vi "Test TDMS.vi"() -> ()   [LabVIEW 2020]
uses:
  Models/Data Types/TDMS/TDMS.lvclass
  Models/Data Types/Abstrut Data/Abstruct Data Type.lvclass/Abstruct Data Type.ctl
  Models/Data Types/Abstrut Data/Accessors/Write File Path.vi
panel:
  in  "Horizontal Pointer Slide 3":cluster{"Numeric":dbl, "Numeric":dbl}(slide)={"Numeric"=0.0, "Numeric"=4.769230769230769} scale=0.0..10.0
  in  "Horizontal Pointer Slide 2":dbl(slide) scale=0.0..10.0
  in  "Horizontal Pointer Slide":cluster{"Numeric":dbl, "Numeric":dbl}(slide)={"Numeric"=0.0, "Numeric"=5.461538461538462} scale=0.0..10.0
  out "Waveform Chart":waveform(dbl)[](graph)
  out "error out":errorcluster
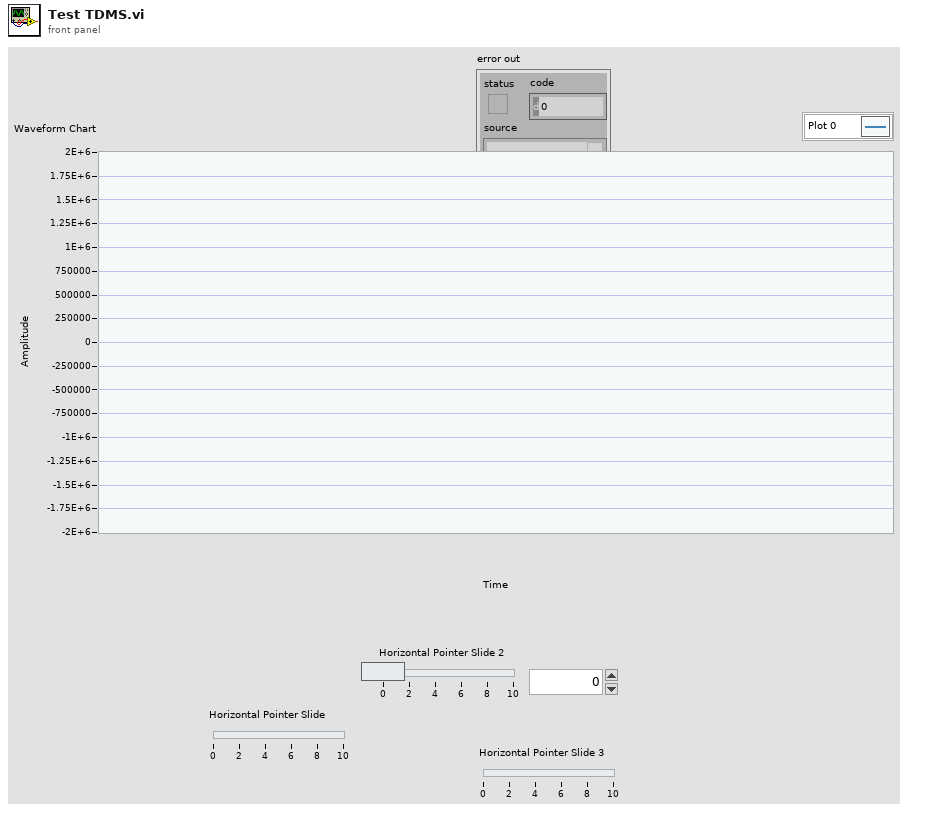
[diagram p1: front panel]
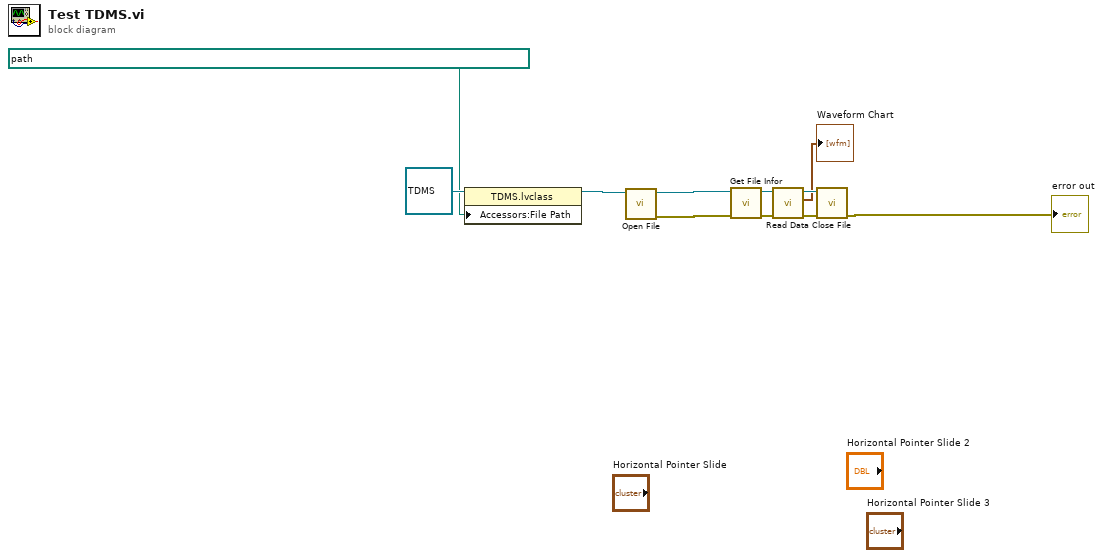
[diagram p0: block diagram]
diagram:
  n1 = property class="TDMS.lvclass"(reference=refnum<class "TDMS.lvclass"> refnum ("TDMS.lvclass"), "Accessors:File Path"=path "D:/13.软件工具/Data View/Source/Test Data/13 Calculate 2022-12-05 15-53-08.629.tdms" ("file path")) -> (reference out=w2:refnum<class "TDMS.lvclass">)  [unwired: 1 in, 1 out]
  n2 = call-dynamic "Open File.vi"("TDMS in"=w2) -> ("error out"=w10:errorcluster, "TDMS out"=w11:refnum<class "TDMS.lvclass">)  [unwired: 9 in]
  n3 = call-dynamic "Get File Infor.vi"("error in (no error)"=w10, "TDMS in"=w11) -> ("error out"=w8:errorcluster, "TDMS out"=w9:refnum<class "TDMS.lvclass">)  [unwired: 8 in]
  n4 = call-dynamic "Read Data.vi"("error in (no error)"=w8, "TDMS in"=w9) -> ("error out"=w6:errorcluster, "data"=→"Waveform Chart":waveform(dbl)[], "TDMS out"=w7:refnum<class "TDMS.lvclass">)  [unwired: 7 in]
  n5 = call-dynamic "Close File.vi"("error in (no error)"=w6, "TDMS in"=w7) -> ("error out"=→"error out":errorcluster)  [unwired: 8 in, 1 out]
